vi "LVPortUpdateObjectMapDataValueToRealNumberOrArrayVariant.vi"(0 "UpdateData":dbl[](array[numeric]), 5 "Sizes":i32[](array[numeric]), 7 "UpdateAt":i32[](array[numeric]), 9 "Has Value":bool, 11 "SourceValue":variant) -> (4 "Value":variant, 8 "Invalid Indexing or errored value":bool)   [LabVIEW 2017]
uses:
  <vilib>/Utility/Data Type/Type Definitions/Data Type.ctl
  <vilib>/Utility/Data Type/NI_Data Type.lvlib
panel:
  out "size(s)":i32
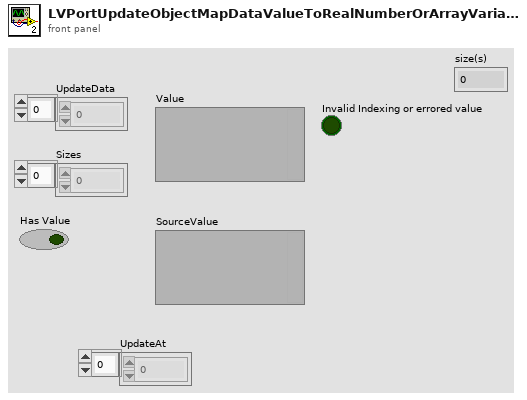
[diagram p1: front panel]
types:
  T1 = typedef "NI_Data Type.lvlib/Data Type.ctl" = enum8{"Invalid Type", "Void", "I8", "I16", "I32", "I64", "U8", "U16", "U32", "U64", "Single Float", "Double Float", "Extended Float", "Single Complex", "Double Complex", "Extended Complex", "Enum U8", "Enum U16", "Enum U32", "Enum U64", "Single Float With Unit", "Double Float With Unit", "Extended Float With Unit", "Single Complex with Unit", "Double Complex with Unit", "Extended Complex with Unit", "Boolean", "String", "Path", "Picture", "Tag", "Array", "Cluster", "Variant", "LV Variant", "Waveform", "Timestamp", "Digital Waveform", "Digital Data", "ExpressData", "Refnum", "External Data", "VI", "Poly VI", "LabVIEW Class Instance", "Fixed Point"}
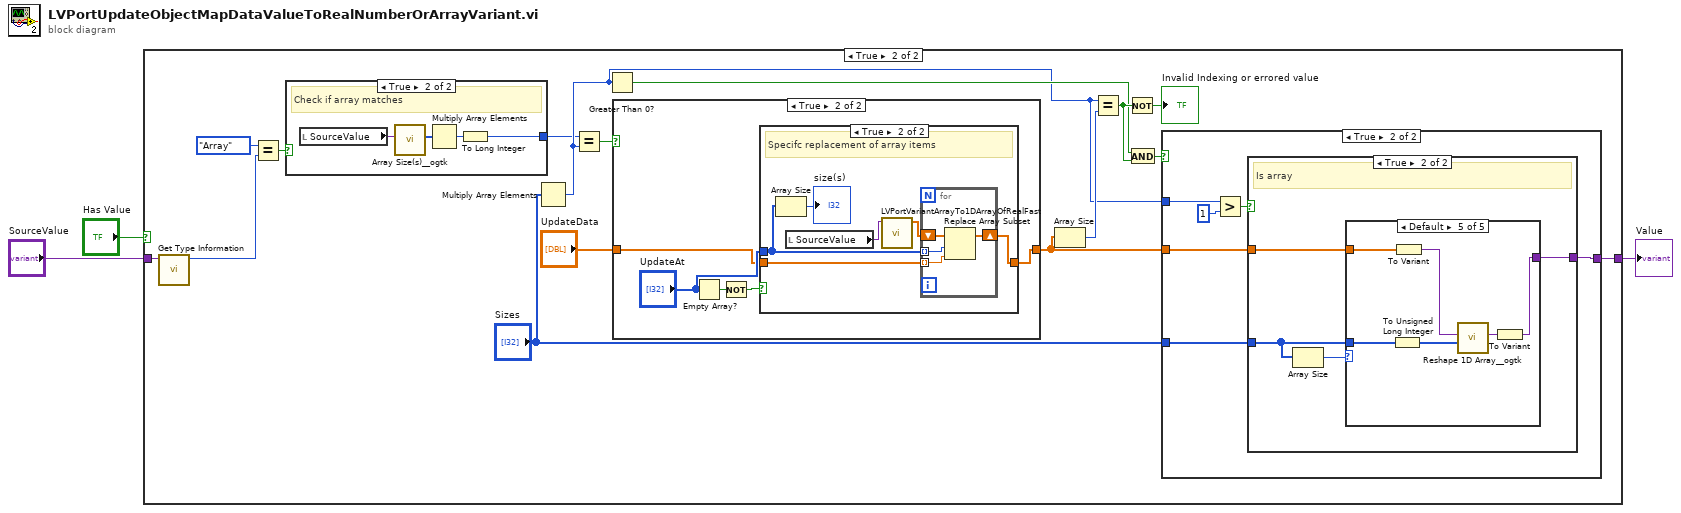
[diagram p0: block diagram]
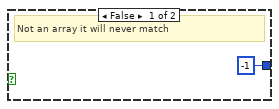
[diagram p3: hidden frame]
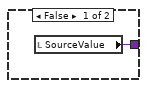
[diagram p6: hidden frame]
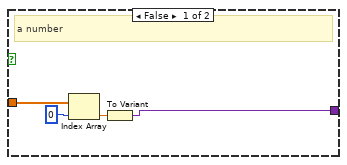
[diagram p7: hidden frame]
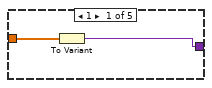
[diagram p8: hidden frame]
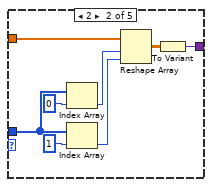
[diagram p9: hidden frame]
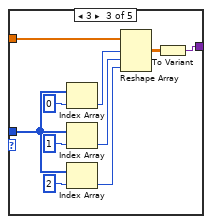
[diagram p10: hidden frame]
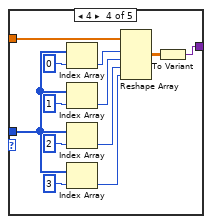
[diagram p11: hidden frame]
diagram:
  n1 = case shown="True" "Has Value" {
    tunnel: [w4 w14] -> w2
    tunnel: "SourceValue" -> [w4 w11]
    frame False {
    }
    frame True {
      n2 = call <vilib>:"Get Type Information.vi"("Variant"=w11) -> ("Type"=w13:T1)  [unwired: 6 in, 4 out]
      n3 = Equal?(x=Data_Type."Array" ("Type"), y=w13) -> (x = y?=w6:bool)
      n4 = case shown="True" w6 {
        tunnel: [-1 w23] -> w7
        frame False {
          # "Not an array it will never match"
        }
        frame True {
          # "Check if array matches"
          n5 = local read "SourceValue"() -> (w22:variant)
          n6 = call <userlib>:"Array Size(s)__ogtk.vi"("Array"=w22) -> ("Size(s)"=w24:u32[])  [unwired: 8 in, 2 out]
          n7 = Multiply Array Elements(1:w24) -> (0:w25:u32)
          n8 = To Long Integer(number=w25) -> (32bit integer=w23:i32)
        }
      }
      n9 = Multiply Array Elements(1:"Sizes") -> (0:w10:i32)
      n10 = Equal?(x=w7, y=w10) -> (x = y?=w9:bool)
      n11 = Greater Than 0?(x=w10) -> (x > 0?=w15:bool)
      n12 = case shown="True" w9 {
        tunnel: [w26 w29] -> w18
        tunnel: "UpdateData" -> [w26 w27]
        frame False {
        }
        frame True {
          n13 = Empty Array?(array="UpdateAt") -> (empty?=w31:bool)
          n14 = Not(x=w31) -> (.not. x?=w30:bool)
          n15 = case shown="True" w30 {
            tunnel: w27 -> [w32 w35]
            tunnel: [w32 w36] -> w29
            tunnel: "UpdateAt" -> [_ w33]
            frame False {
              # "The new array is the new value"
            }
            frame True {
              # "Specifc replacement of array items"
              n16 = Array Size(array=w33) -> (size(s)=→"size(s)":i32)
              n17 = local read "SourceValue"() -> (w37:variant)
              n18 = call "LVPortVariantArrayTo1DArrayOfRealFast.vi"("Variant Real Array"=w37) -> ("1D Array"=w38:dbl[])  [unwired: 8 in, 2 out]
              n19 = for {
                shift-right: [w39] -> w36
                shift-left: w38 -> [w42]
                tunnel: w35 -> [w41] mode=indexing
                tunnel: w33 -> [w40] mode=indexing
                n20 = Replace Array Subset(array=w42, new element=w41, index=w40) -> (w39:dbl[])
              }
            }
          }
        }
      }
      n21 = Array Size(array=w18) -> (size(s)=w17:i32)
      n22 = Equal?(x=w10, y=w17) -> (x = y?=w16:bool)
      n23 = Not(x=w16) -> (.not. x?=→"Invalid Indexing or errored value":bool)
      n24 = And(x=w15, y=w16) -> (x .and. y?=w19:bool)
      n25 = case shown="True" w19 {
        tunnel: "Sizes" -> [_ w46]
        tunnel: w18 -> [_ w47]
        tunnel: [w43 w45] -> w14
        tunnel: w10 -> [_ w49]
        frame False {
          n26 = local read "SourceValue"() -> (w43:variant)
        }
        frame True {
          n27 = Greater?(x=w49, y=1) -> (0:w48:bool)
          n28 = case shown="True" w48 {
            tunnel: w47 -> [w53 w55]
            tunnel: w46 -> [_ w54]
            tunnel: [w50 w56] -> w45
            frame False {
              # "a number"
              n29 = Index Array(array=w53, index=0) -> (element=w51:dbl)
              n30 = To Variant(anything=w51) -> (Variant=w50:variant)
            }
            frame True {
              # "Is array"
              n31 = Array Size(array=w54) -> (size(s)=w57:i32)
              n32 = case shown="Default" w57 {
                tunnel: [w58 w60 w68 w78 w94] -> w56
                tunnel: w55 -> [w59 w67 w73 w83 w90]
                tunnel: w54 -> [_ w66 w71 w81 w93]
                frame 1 {
                  n33 = To Variant(anything=w59) -> (Variant=w58:variant)
                }
                frame 2 {
                  n34 = Index Array(array=w66, index=0) -> (element=w65:i32)
                  n35 = Index Array(array=w66, index=1) -> (element=w64:i32)
                  n36 = Reshape Array(w67, w65, w64) -> (w61:dbl[][])
                  n37 = To Variant(anything=w61) -> (Variant=w60:variant)
                }
                frame 3 {
                  n38 = Index Array(array=w71, index=0) -> (element=w77:i32)
                  n39 = Index Array(array=w71, index=1) -> (element=w76:i32)
                  n40 = Index Array(array=w71, index=2) -> (element=w70:i32)
                  n41 = Reshape Array(w73, w77, w76, w70) -> (w69:dbl[][][])
                  n42 = To Variant(anything=w69) -> (Variant=w68:variant)
                }
                frame 4 {
                  n43 = Index Array(array=w81, index=0) -> (element=w89:i32)
                  n44 = Index Array(array=w81, index=1) -> (element=w88:i32)
                  n45 = Index Array(array=w81, index=2) -> (element=w84:i32)
                  n46 = Index Array(array=w81, index=3) -> (element=w80:i32)
                  n47 = Reshape Array(w83, w89, w88, w84, w80) -> (w79:dbl[][][][])
                  n48 = To Variant(anything=w79) -> (Variant=w78:variant)
                }
                frame Default {
                  n49 = To Unsigned Long Integer(number=w93) -> (unsigned 32bit integer=w92:u32[])
                  n50 = To Variant(anything=w90) -> (Variant=w91:variant)
                  n51 = call <userlib>:"Reshape 1D Array__ogtk.vi"("Size(s)"=w92, "1D Array"=w91) -> ("Reshaped VArray"=w95:variant)  [unwired: 8 in, 1 out]
                  n52 = To Variant(anything=w95) -> (Variant=w94:variant)
                }
              }
            }
          }
        }
      }
    }
  }
  "Value" <- w2
